vi "Byte Buffer.Destroy.vi"(8 "error in (no error)":errorcluster, 11 "Byte Buffer in":refnum<class "Byte Buffer.lvclass">) -> (0 "error out":errorcluster)   [LabVIEW 2016, in "VeriStand Data.lvlib" / "Byte Buffer.lvclass"]
doc: "Destroys all pointers associated with the provided <B>Byte Buffer</B>."
uses:
  Byte Buffer.lvclass
  Byte Buffer.lvclass/Byte Buffer.ctl
  VeriStand Data.lvlib
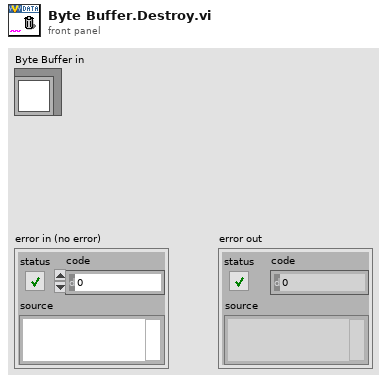
[diagram p1: front panel]
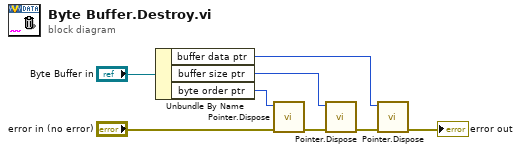
[diagram p0: block diagram]
diagram:
  n1 = Unbundle By Name("Byte Buffer in") -> ("buffer data ptr"=w1:u64, "buffer size ptr"=w2:u64, "byte order ptr"=w3:u64)
  n2 = call "Pointer.Dispose.vi"("error in (no error)"="error in (no error)", "pointer"=w3) -> ("error out"=w6:errorcluster)  [unwired: 8 in, 1 out]
  n3 = call "Pointer.Dispose.vi"("error in (no error)"=w6, "pointer"=w2) -> ("error out"=w5:errorcluster)  [unwired: 8 in, 1 out]
  n4 = call "Pointer.Dispose.vi"("error in (no error)"=w5, "pointer"=w1) -> ("error out"=→"error out":errorcluster)  [unwired: 8 in, 1 out]
